vi "Software Update HCC Archive Folder Creation.vi"(7 "Numeric":i32, 8 "Error In":errorcluster, 9 "Newfi Exe Folder Path":path=path "C:/Newfi Exe", 11 "Path Build List Sub":path) -> (0 "Error Out":errorcluster, 1 "folder names":string[](array[string]))   [LabVIEW 2016]
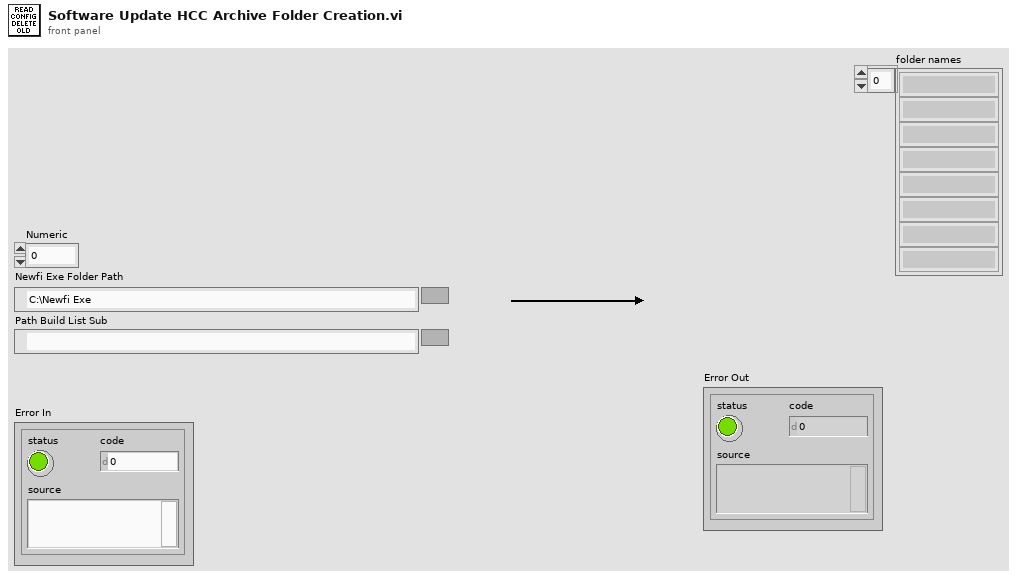
[diagram p1: front panel]
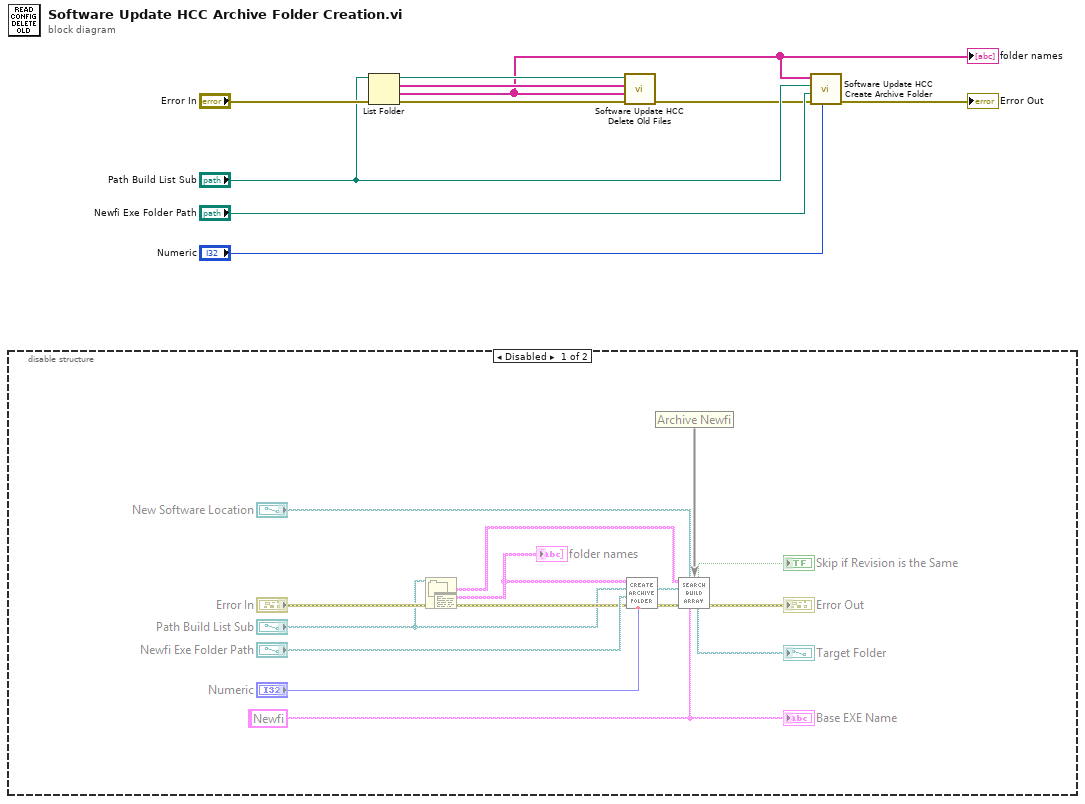
[diagram p0: block diagram]
diagram:
  n1 = disable-structure shown="Disabled" {
    frame Disabled {
    }
    frame Enabled {
    }
  }
  n2 = List Folder(path="Path Build List Sub", error in="Error In") -> (filenames=w2:string[], folder names=w1:string[], error out=w4:errorcluster)  [unwired: 2 in, 1 out]
  "folder names" <- w1
  n3 = call "Software Update HCC Delete Old Files.vi"("Error In"=w4, "folder names"=w1, "filenames"=w2, "Path Build List Sub"="Path Build List Sub") -> ("Error Out"=w3:errorcluster)  [unwired: 7 in]
  n4 = call "Software Update HCC Create Archive Folder.vi"("Station Location (Index)"="Numeric", "error in (no error)"=w3, "Newfi Exe Folder Path"="Newfi Exe Folder Path", "Path"="Path Build List Sub", "folder names"=w1) -> ("error out"=→"Error Out":errorcluster)  [unwired: 5 in, 1 out]
